vi "Launcher.vi"() -> ()   [LabVIEW 2017, in "Actor Example.lvlib"]
uses:
  Actor Example.lvlib
  Actor Example/Actor Example.lvclass
  C:/Program Files (x86)/National Instruments/LabVIEW 2017/vi.lib/ActorFramework/Actor/Actor.lvclass
  Actor Example/Actor Example.lvclass/Actor Example.ctl
  Actor Example Messages/Start Long Running Process Msg/Start Long Running Process Msg.lvclass/Start Long Running Process Msg.ctl
  <vilib>/ActorFramework/Message Enqueuer/Message Enqueuer.lvclass/Message Enqueuer.ctl
  9016dfb5-e5ce-4350-9d9b-bb4e643018af.vi
  6511bd4d-de14-4cd5-9039-b7c5838a1cf0.vi
  Actor Example/Write Threshold.vi
  <vilib>/ActorFramework/Message Enqueuer/Enqueue.vi
  Actor Example Messages/Start Long Running Process Msg/Start Long Running Process Msg.lvclass
  C:/Program Files (x86)/National Instruments/LabVIEW 2017/vi.lib/ActorFramework/Message/Message.lvclass
  <vilib>/ActorFramework/Stop Msg/Stop Msg.lvclass
  Promise Future/Promise/Obtain Promise.vi
  <vilib>/ActorFramework/Message Priority Queue/Priority Enqueue.vi
  Actor Example Callback.vi
  Promise Future/Future/Wrapper VI Name.vi
  Promise Future/Future/Then.vi
  Promise Future/Future/Read Future.vi
  <vilib>/ActorFramework/Actor/Actor.lvclass
panel:
  out "Value":dbl format="%#_13g"
  in  "Threshold":dbl=0.2 format="%#_13g"
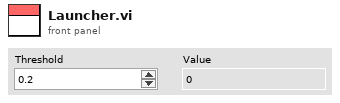
[diagram p1: front panel]
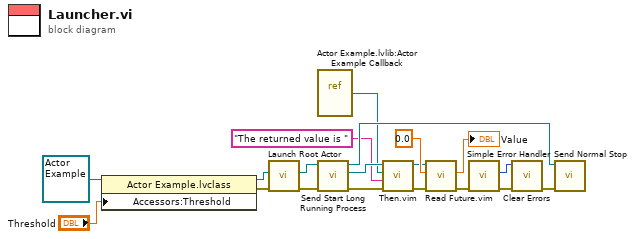
[diagram p0: block diagram]
diagram:
  n1 = property class="Actor Example.lvclass"(reference=refnum<class "Actor Example.lvclass"> refnum ("Actor Example.lvlib:Actor Example.lvclass"), "Accessors:Threshold"="Threshold") -> (reference out=w16:refnum<class "Actor Example.lvclass">, error out=w15:errorcluster)  [unwired: 1 in]
  n2 = call <vilib>:"Launch Root Actor.vi"("error in (no error)"=w15, "Actor"=w16) -> ("error out"=w18:errorcluster, "Actor's Enqueuer"=w19:refnum<class "Message Enqueuer.lvclass">)  [unwired: 8 in]
  n3 = vi-ref "Actor Example.lvlib:Actor Example Callback.vi"() -> (w1:refnum<vi>)
  n4 = call "Send Start Long Running Process.vi"("error in (no error)"=w18, "Message Enqueuer"=w19) -> ("error out"=w4:errorcluster, "Future"=w3:refnum<class "Future.lvclass">, "Message Enqueuer out"=w13:refnum<class "Message Enqueuer.lvclass">)  [unwired: 7 in]
  n5 = call "Then.vim"("error in (no error)"=w4, "Scope"="The returned value is ", "VI"=w1, "Future in"=w3) -> ("error out"=w5:errorcluster, "Future out"=w6:refnum<class "Future.lvclass">)  [unwired: 6 in]
  n6 = call "Read Future.vim"("error in (no error)"=w5, "Default Value"=0.0 ("Threshold"), "Future in"=w6) -> ("error out"=w7:errorcluster, "Value"=→"Value":dbl)  [unwired: 5 in, 2 out]
  n7 = call <vilib>:"Simple Error Handler.vi"("error in (no error)"=w7) -> ("code out"=w11:i32, "error out"=w12:errorcluster)  [unwired: 4 in, 3 out]
  n8 = call <vilib>:"Clear Errors.vi"("error in (no error)"=w12, "specific error code to clear (0: all)"=w11) -> ("error out"=w10:errorcluster)  [unwired: 4 in, 1 out]
  n9 = call <vilib>:"Send Normal Stop.vi"("error in (no error)"=w10, "Message Enqueuer"=w13) -> ()  [unwired: 9 in, 1 out]
